vi "对话框模板.vi"(8 "error in (no error)":errorcluster, 9 "message":string, 11 "Window Title (\"\")":string) -> (0 "error out":errorcluster, 2 "Which Button?":T1(ring)=enum."Center Button")   [LabVIEW 2015]
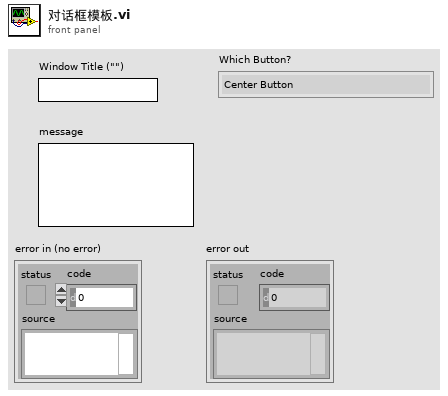
[diagram p1: front panel]
types:
  T1 = enum16{"Left Button", "Center Button", "Right Button", "Window Close"}
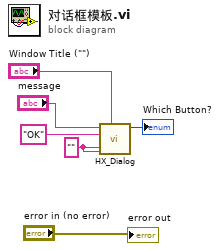
[diagram p0: block diagram]
diagram:
  w6 = "" ("Center Button Text (\"No\")")
  n1 = call "HX_Dialog.vi"("Window Title (\"\")"="Window Title (\"\")", "Right Button Text (\"Cancel\")"=w6, "Center Button Text (\"No\")"=w6, "Left Button Text (\"Yes\")"="OK" ("Left Button Text (\"Yes\")"), "message"="message") -> ("Which Button?"=→"Which Button?":T1)  [unwired: 6 in]
  "error out" <- "error in (no error)"
